vi "runTestScenario.vi"(0 "Digital Input Test  in":refnum<class "Test Pressure.lvclass">, 5 "ILC":refnum<class "ILC.lvclass">, 11 "error in (no error)":errorcluster) -> (4 "Digital Input Test out":refnum<class "Test Pressure.lvclass">, 6 "ILC 2":refnum<class "ILC.lvclass">, 8 "TestExecution":T2, 10 "Result":T1, 15 "error out":errorcluster)   [LabVIEW 2015, in "Test Pressure.lvclass"]
uses:
  Test Pressure.lvclass
  Typedefs/TestExecution.ctl
  Typedefs/PassFailTest.ctl
  <userlib>/Common/ILC/ILC/ILC.lvclass
  Typedefs/WriteLogMessageInput.ctl
  Typedefs/TestScenarioTypes.ctl
  Typedefs/WriteDataFileInput.ctl
  Test Pressure.lvclass/Test Pressure.ctl
  Model/TestLog/ITestLog/ITestLog.lvclass
  Model/ConfigureILCStrategy/IConfigureILCStrategy/IConfigureILCStrategy.lvclass
  Model/ReadILCStrategy/IReadILCStrategy/IReadILCStrategy.lvclass
  Typedefs/ILCBTTypedefs.lvlib
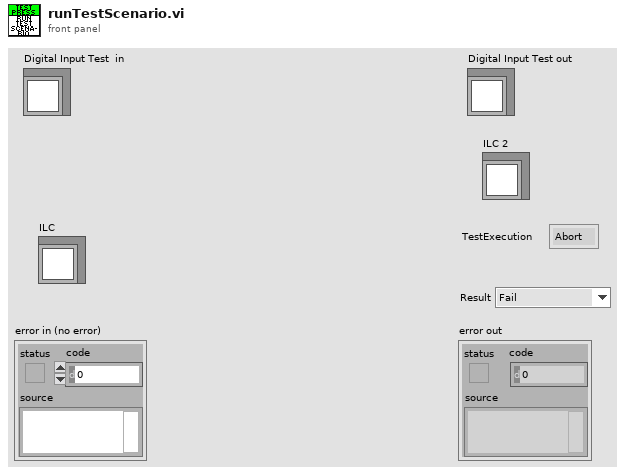
[diagram p1: front panel]
types:
  T1 = typedef "ILCBTTypedefs.lvlib/PassFailTest.ctl" = enum16{"Fail", "Pass", "NA"}
  T2 = typedef "ILCBTTypedefs.lvlib/TestExecution.ctl" = enum16{"Abort", "Continue"}
  T3 = typedef "ILCBTTypedefs.lvlib/WriteDataFileInput.ctl" = cluster{"Test Scenario":T4, "File Name":string, "Output":string[]}
  T4 = typedef "ILCBTTypedefs.lvlib/TestScenarioTypes.ctl" = enum16{"+3.3VD", "+5.1V", "+24V", "RELVALV1", "RELVALV2", "Verify DAC_A = -1.00A", "Verify DAC_A = -0.75A", "Verify DAC_A = -0.50A", "Verify DAC_A = -0.25A", "Verify DAC_A = 0.00A", "Verify DAC_A = 0.25A", "Verify DAC_A = 0.50A", "Verify DAC_A = 0.75A", "Verify DAC_A = 1.00A", "Verify DAC_B = -1.00A", "Verify DAC_B = -0.75A", "Verify DAC_B = -0.50A", "Verify DAC_B = -0.25A", "Verify DAC_B = 0.00A", "Verify DAC_B = 0.25A", "Verify DAC_B = 0.50A", "Verify DAC_B = 0.75A", "Verify DAC_B = 1.00A", "Set DAC_A = -1.00A", "Set DAC_A = -0.75A", "Set DAC_A = -0.50A", "Set DAC_A = -0.25A", "Set DAC_A = 0.00A", "Set DAC_A = 0.25A", "Set DAC_A = 0.50A", "Set DAC_A = 0.75A", "Set DAC_A = 1.00A", "Set DAC_B = -1.00A", "Set DAC_B = -0.75A", "Set DAC_B = -0.50A", "Set DAC_B = -0.25A", "Set DAC_B = 0.00A", "Set DAC_B = 0.25A", "Set DAC_B = 0.50A", "Set DAC_B = 0.75A", "Set DAC_B = 1.00A", "Set MTR_PWR = On", "Set MTR_PWR = Off", "Set OUTPUT = On", "Set OUTPUT = Off", "Verify OUTPUT = On", "Verify OUTPUT = Off", "Verify POWER = Ok", "Verify POWER = Fail", "Verify AMP1 = Ok", "Verify AMP1 = Fail", "Verify AMP2 = Ok", "Verify AMP2 = Fail", "P1 0%", "P1 25%", "P1 50%", "P1 75%", "P1 100%", "P2 0%", "P2 25%", "P2 50%", "P2 75%", "P2 100%", "P3 0%", "P3 25%", "P3 50%", "P3 75%", "P3 100%", "P4 0%", "P4 25%", "P4 50%", "P4 75%", "P4 100%"}
  T5 = typedef "ILCBTTypedefs.lvlib/WriteLogMessageInput.ctl" = cluster{"Test Scenario":T4, "Description":string, "Actual Value":string, "Data File":string, "Result":T1}
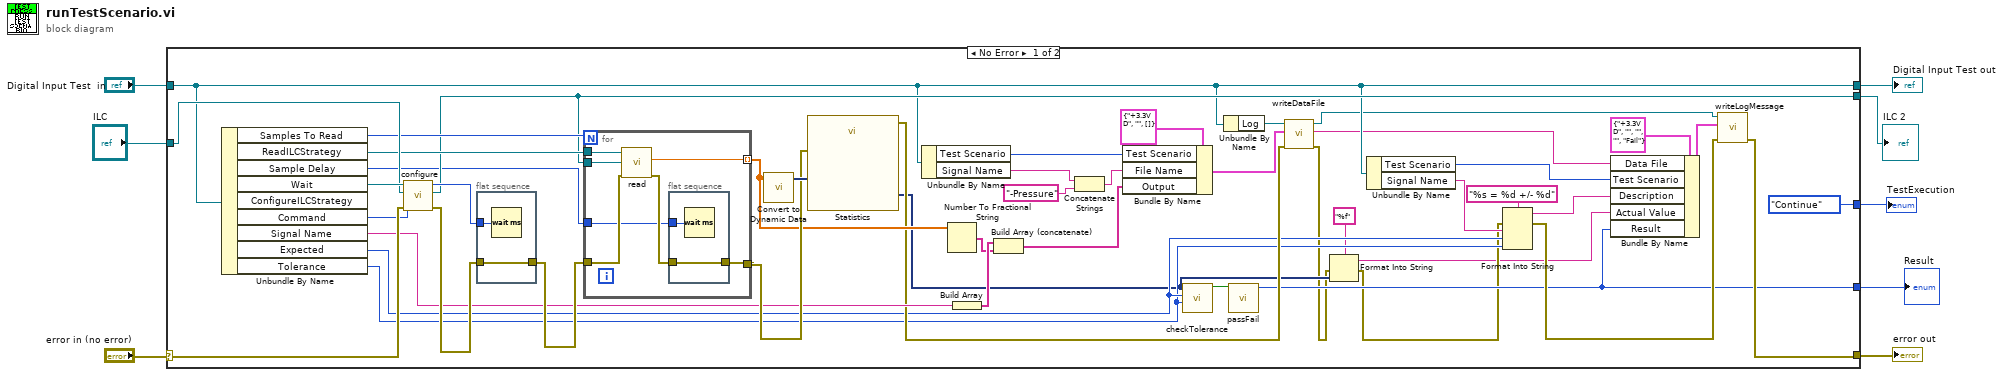
[diagram p0: block diagram]
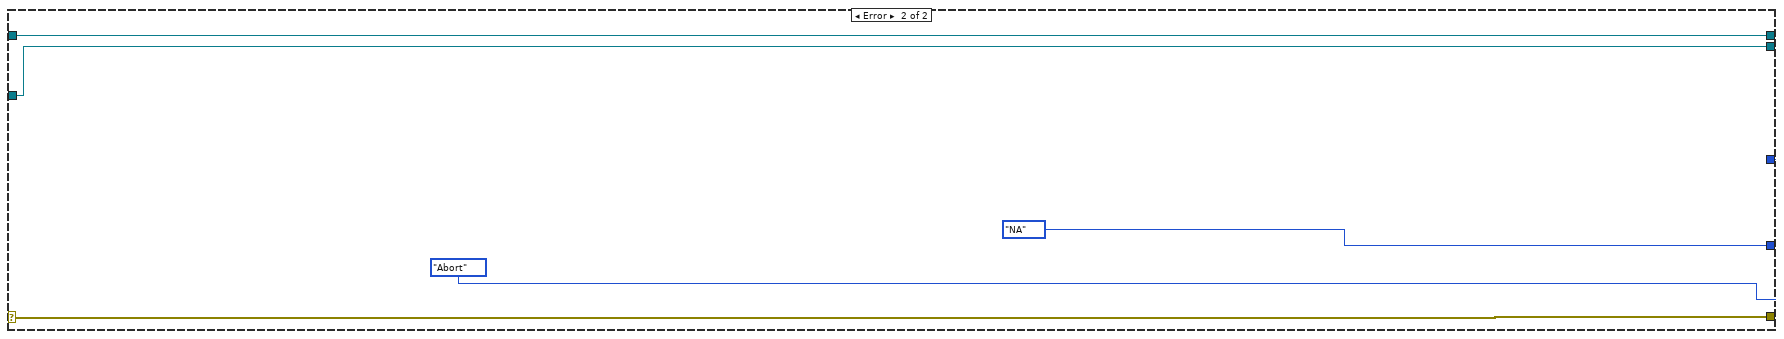
[diagram p2: hidden frame]
diagram:
  n1 = case shown="No Error" "error in (no error)" {
    selector: "error in (no error)" -> [w46 w71]
    tunnel: [w55 w71] -> w7
    tunnel: [TestExecution."Continue" ("TestExecution") TestExecution."Abort" ("TestExecution")] -> w6
    tunnel: "Digital Input Test  in" -> [w23 w69]
    tunnel: [w23 w69] -> w4
    tunnel: "ILC" -> [w41 w68]
    tunnel: [w16 PassFailTest."NA" ("Result")] -> w2
    tunnel: [w37 w68] -> w1
    frame No Error {
      n2 = Unbundle By Name(w23) -> ("Samples To Read"=w40:i32, "ReadILCStrategy"=w39:refnum<class "IReadILCStrategy.lvclass">, "Sample Delay"=w36:i32, "Wait"=w42:i32, "ConfigureILCStrategy"=w53:refnum<class "IConfigureILCStrategy.lvclass">, "Command"=w45:u16, "Signal Name"=w33:string, "Expected"=w15:u16, "Tolerance"=w14:u16)
      n3 = call-dynamic "configure.vi"("error in (no error)"=w46, "Value"=w45, "ILC"=w41, "IConfigureILCStrategy in"=w53) -> ("error out"=w43:errorcluster, "ILC 2"=w37:refnum<class "ILC.lvclass">)  [unwired: 5 in, 1 out]
      n4 = flat-sequence {
        tunnel: w43 -> [w66]
        tunnel: [w66] -> w38
        tunnel: w42 -> [w65]
        frame #0 {
          n5 = Wait (ms)(milliseconds to wait=w65) -> ()  [unwired: 1 out]
        }
      }
      n6 = for {
        N: w40 -> [_]
        tunnel: w39 -> [w62]
        tunnel: [w61] -> w34
        tunnel: w38 -> [w60]
        tunnel: w37 -> [w58]
        tunnel: [w57] -> w30 mode=indexing
        tunnel: w36 -> [w56]
        n7 = call-dynamic "read.vi"("error in (no error)"=w60, "ILC"=w58, "IReadILCStrategy in"=w62) -> ("error out"=w59:errorcluster, "Value"=w57:dbl)  [unwired: 6 in, 1 out]
        n8 = flat-sequence {
          tunnel: w59 -> [w64]
          tunnel: [w64] -> w61
          tunnel: w56 -> [w63]
          frame #0 {
            n9 = Wait (ms)(milliseconds to wait=w63) -> ()  [unwired: 1 out]
          }
        }
      }
      n10 = call "Convert to Dynamic Data"("Array"=w30) -> ("Dynamic Data Type"=w35:dynamicdata)  [unwired: 3 in]
      n11 = call "Statistics"("Signals"=w35, "error in (no error)"=w34) -> ("Arithmetic Mean"=w13:dynamicdata, "error out"=w20:errorcluster)  [unwired: 24 in]
      n12 = Unbundle By Name(w23) -> ("Test Scenario"=w28:T4, "Signal Name"=w25:string)
      n13 = Number To Fractional String(number=w30) -> (F-format string=w31:string[])  [unwired: 3 in]
      n14 = Build Array(w33) -> (w32:string[])
      n15 = Build Array (concatenate)(w32, w31) -> (w24:string[])
      n16 = Concatenate Strings(w25, "-Pressure" ("string")) -> (w26:string)
      n17 = Bundle By Name(cluster=T3 {"Test Scenario"=enum."+3.3VD", "File Name"="", "Output"=[]} ("WriteDataFileInput"), "Test Scenario"=w28, "File Name"=w26, "Output"=w24) -> (w21:T3)
      n18 = call "checkTolerance.vi"("Tolerance"=w14, "Expected Value"=w15, "Average"=w13) -> ("Boolean"=w17:bool)  [unwired: 8 in]
      n19 = Unbundle By Name(w23) -> ("Log"=w22:refnum<class "ITestLog.lvclass">)
      n20 = call "passFail.vi"("Boolean"=w17) -> ("Result"=w16:T1)  [unwired: 10 in]
      n21 = call-dynamic "writeDataFile.vi"("error in (no error)"=w20, "WriteDataFileInput"=w21, "ITestLog in"=w22) -> ("error out"=w11:errorcluster, "Relative Path"=w19:string, "ITestLog out"=w18:refnum<class "ITestLog.lvclass">)  [unwired: 6 in]
      n22 = Format Into String(format string="%f", error in=w11, w13) -> (resulting string=w9:string, error out=w10:errorcluster)  [unwired: 1 in]
      n23 = Unbundle By Name(w23) -> ("Test Scenario"=w48:T4, "Signal Name"=w52:string)
      n24 = Format Into String(format string="%s = %d +/- %d", error in=w10, w52, w15, w14) -> (resulting string=w49:string, error out=w44:errorcluster)  [unwired: 1 in]
      n25 = Bundle By Name(cluster=T5 {"Test Scenario"=enum."+3.3VD", "Description"="", "Actual Value"="", "Data File"="", "Result"=enum."Fail"} ("WriteLogMessageInput"), "Data File"=w19, "Test Scenario"=w48, "Description"=w49, "Actual Value"=w9, "Result"=w16) -> (w50:T5)
      n26 = call-dynamic "writeLogMessage.vi"("error in (no error)"=w44, "WriteLogMessageInput"=w50, "ITestLog in"=w18) -> ("error out"=w55:errorcluster)  [unwired: 7 in, 1 out]
    }
    frame Error {
    }
  }
  "Digital Input Test out" <- w4
  "error out" <- w7
  "TestExecution" <- w6
  "Result" <- w2
  "ILC 2" <- w1
